vi "ScanningWaveformline_v1.vi"(0 "Vx-max":dbl, 1 "linepixels":dbl, 5 "Vx-min":dbl, 7 "AOrate":dbl, 9 "Vy-max":dbl, 11 "Vy-min":dbl, 12 "numlines":dbl) -> (3 "X-WaveArray":dbl[](array[numeric]), 6 "numPixels":dbl, 14 "Y-WaveArray":dbl[](array[numeric]), 15 "P":dbl)   [LabVIEW 2013]
panel:
  out "flyback time y (us)":dbl
  out "flyback time x (us)":dbl
  out "Waveform Graph 2":dbl[](graph)
  out "Waveform Graph":dbl[](graph)
  out "C":dbl
  out "S":dbl
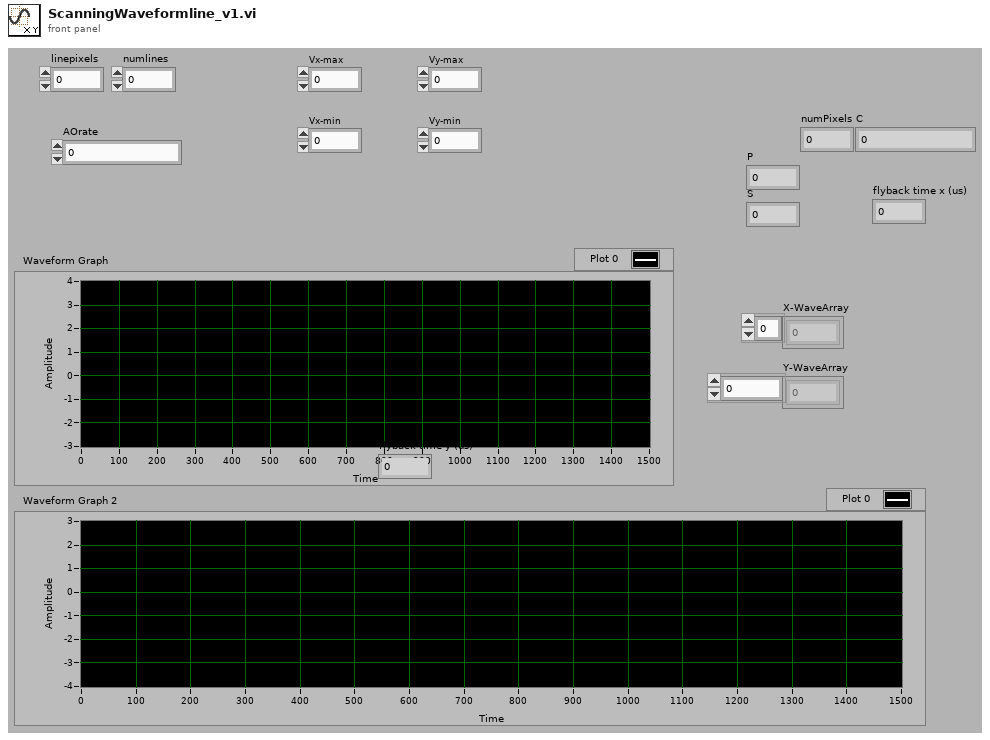
[diagram p1: front panel]
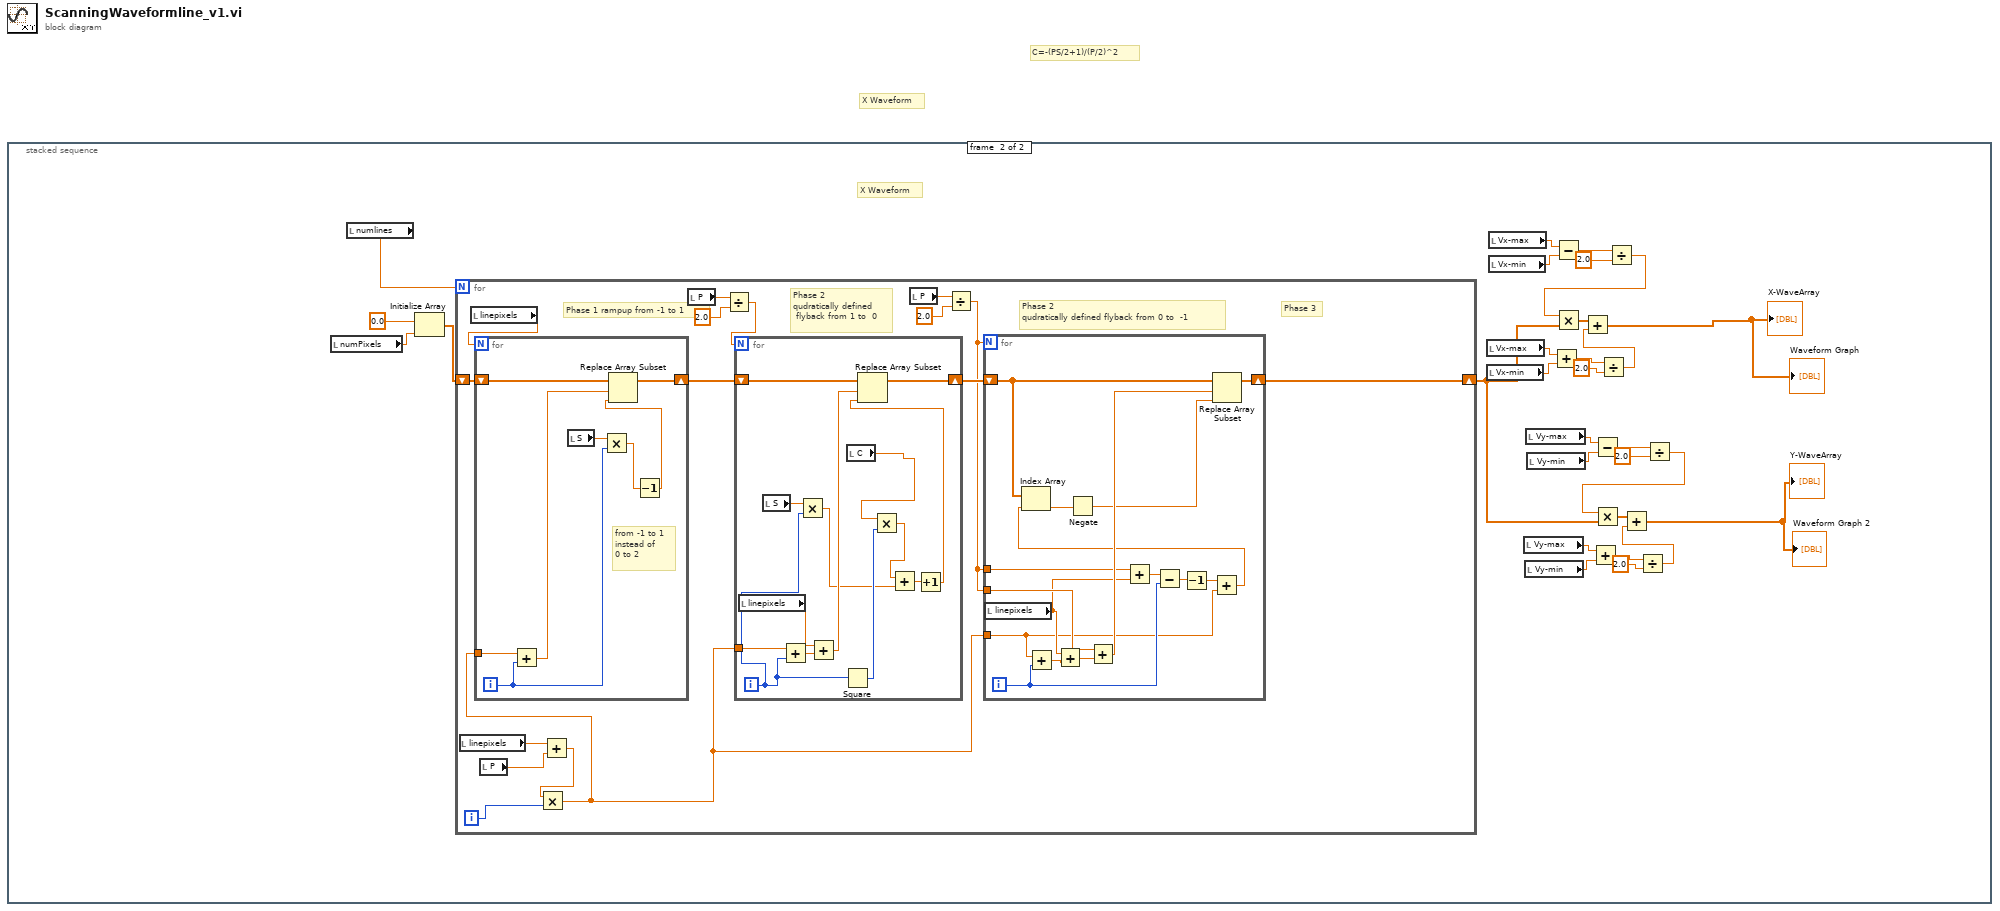
[diagram p0: block diagram]
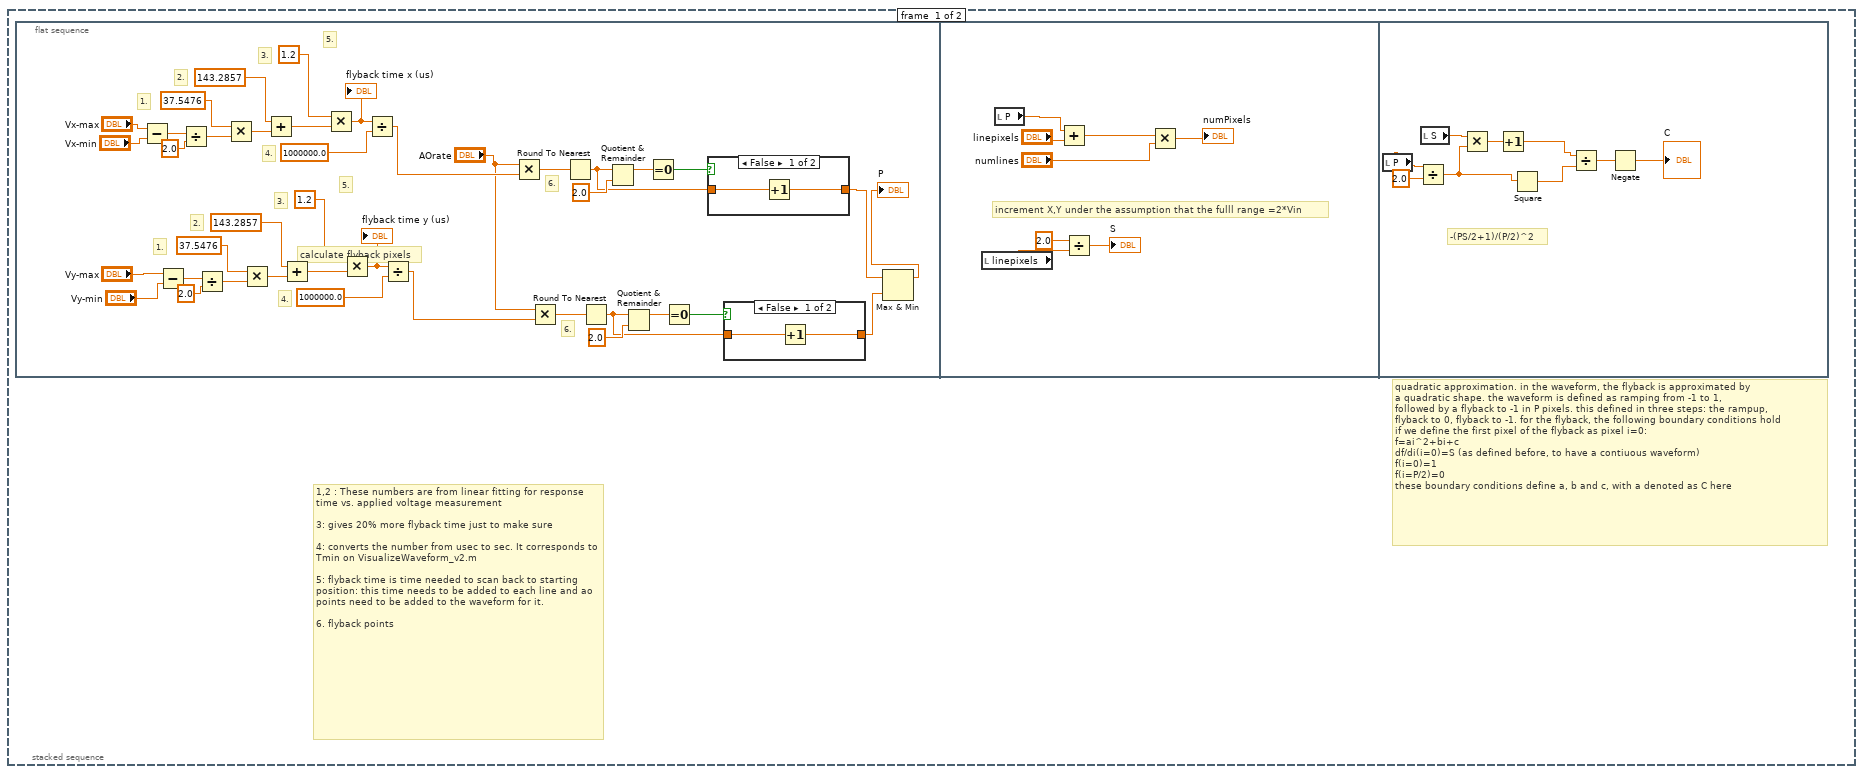
[diagram p2: hidden frame]
diagram:
  # "C=-(PS/2+1)/(P/2)^2"
  # "X Waveform"
  n1 = stacked-sequence {
    frame #0 {
      # "quadratic approximation. in the waveform, the flyback is approximated by\na quadratic shape. the waveform is defined as ramping from -1 to 1, \nfollowed by a flyback to -1 in P pixels. this defined in three steps: the rampup,\nflyback to 0, flyback to -1. for the flyback, the following boundary conditions hold\nif we define the first pixel of the flyback as pixel i=0:\nf=ai^2+bi+c\ndf/di(i=0)=S (as defined before, to have a contiuous waveform)\nf(i=0)=1\nf(i=P/2)=0\nthese boundary conditions define a, b and c, with a denoted as C here"
      # "1,2 : These numbers are from linear fitting for response time vs. applied voltage measurement\n\n3: gives 20% more flyback time just to make sure\n\n4: converts the number from usec to sec. It corresponds to Tmin on VisualizeWaveform_v2.m\n\n5: flyback time is time needed to scan back to starting position: this time needs to be added to each line and ao points need to be added to the waveform for it.\n\n6. flyback points"
      n2 = flat-sequence {
        frame #0 {
          # "6."
          # "5."
          # "4."
          # "3."
          # "2."
          # "1."
          # "calculate flyback pixels"
          # "6."
          # "5."
          # "4."
          # "3."
          # "2."
          # "1."
          n3 = Subtract(x="Vx-max", y="Vx-min") -> (x-y=w24:dbl)
          n4 = Subtract(x="Vy-max", y="Vy-min") -> (x-y=w8:dbl)
          n5 = Divide(x=w24, y=2.0 ("x-y")) -> (x/y=w23:dbl)
          n6 = Divide(x=w8, y=2.0 ("x-y")) -> (x/y=w7:dbl)
          n7 = Multiply(x=37.5476, y=w23) -> (x*y=w39:dbl)
          n8 = Multiply(x=37.5476, y=w7) -> (x*y=w21:dbl)
          n9 = Add(x=143.2857, y=w39) -> (x+y=w37:dbl)
          n10 = Add(x=143.2857, y=w21) -> (x+y=w19:dbl)
          n11 = Multiply(x=1.2, y=w37) -> (x*y=w35:dbl)
          "flyback time x (us)" <- w35
          n12 = Multiply(x=1.2, y=w19) -> (x*y=w17:dbl)
          "flyback time y (us)" <- w17
          n13 = Divide(x=w35, y=1000000.0 ("x")) -> (x/y=w33:dbl)
          n14 = Divide(x=w17, y=1000000.0 ("x")) -> (x/y=w15:dbl)
          n15 = Multiply(x="AOrate", y=w33) -> (x*y=w32:dbl)
          n16 = Multiply(x="AOrate", y=w15) -> (x*y=w14:dbl)
          n17 = Round To Nearest(number=w32) -> (nearest integer value=w28:dbl)
          n18 = Round To Nearest(number=w14) -> (nearest integer value=w10:dbl)
          n19 = Quotient & Remainder(x=w28, y=2.0) -> (x-y*floor(x/y)=w29:dbl)  [unwired: 1 out]
          n20 = Quotient & Remainder(x=w10, y=2.0) -> (x-y*floor(x/y)=w11:dbl)  [unwired: 1 out]
          n21 = Equal To 0?(x=w29) -> (x = 0?=w30:bool)
          n22 = Equal To 0?(x=w11) -> (x = 0?=w12:bool)
          n23 = case shown="False" w30 {
            tunnel: [w44 w46] -> w4
            tunnel: w28 -> [w45 w46]
            frame False {
              n24 = Increment(x=w45) -> (x+1=w44:dbl)
            }
            frame True {
            }
          }
          n25 = case shown="False" w12 {
            tunnel: [w41 w43] -> w5
            tunnel: w10 -> [w42 w43]
            frame False {
              n26 = Increment(x=w42) -> (x+1=w41:dbl)
            }
            frame True {
            }
          }
          n27 = Max & Min(x=w4, y=w5) -> (max(x,y)=→"P":dbl)  [unwired: 1 out]
        }
        frame #1 {
          # "increment X,Y under the assumption that the fulll range =2*Vin"
          n28 = local read "linepixels"() -> (w48:dbl)
          n29 = local read "P"() -> (w54:dbl)
          n30 = Add(x=w54, y="linepixels") -> (x+y=w50:dbl)
          n31 = Divide(x=2.0, y=w48) -> (x/y=→"S":dbl)
          n32 = Multiply(x=w50, y="numlines") -> (x*y=→"numPixels":dbl)
        }
        frame #2 {
          # "-(PS/2+1)/(P/2)^2"
          n33 = local read "P"() -> (w61:dbl)
          n34 = Divide(x=w61, y=2.0) -> (x/y=w63:dbl)
          n35 = local read "S"() -> (w62:dbl)
          n36 = Multiply(x=w62, y=w63) -> (x*y=w58:dbl)
          n37 = Increment(x=w58) -> (x+1=w55:dbl)
          n38 = Square(x=w63) -> (x^2=w59:dbl)
          n39 = Divide(x=w55, y=w59) -> (x/y=w60:dbl)
          n40 = Negate(x=w60) -> (-x=→"C":dbl)
        }
      }
    }
    frame #1 {
      # "X Waveform"
      n41 = local read "numPixels"() -> (w90:dbl)
      n42 = local read "numlines"() -> (w92:dbl)
      n43 = Initialize Array(0.0 ("element"), w90) -> (w89:dbl[])
      n44 = for {
        N: w92 -> [_]
        shift-right: [w94] -> w65
        shift-left: w89 -> [w103]
        i -> [w108]
        # "Phase 2\nqudratically defined flyback from 0 to  -1"
        # "Phase 3"
        # "Phase 2\nqudratically defined\n flyback from 1 to  0"
        # "Phase 1 rampup from -1 to 1"
        n45 = local read "linepixels"() -> (w107:dbl)
        n46 = local read "linepixels"() -> (w104:dbl)
        n47 = local read "P"() -> (w106:dbl)
        n48 = Add(x=w107, y=w106) -> (x+y=w105:dbl)
        n49 = Multiply(x=w105, y=w108) -> (x*y=w93:dbl)
        n50 = for {
          N: w104 -> [_]
          shift-right: [w140] -> w95
          shift-left: w103 -> [w146]
          tunnel: w93 -> [w139]
          i -> [w143]
          # "from -1 to 1\ninstead of\n0 to 2"
          n51 = Add(x=w139, y=w143) -> (x+y=w145:dbl)
          n52 = local read "S"() -> (w144:dbl)
          n53 = Multiply(x=w144, y=w143) -> (x*y=w142:dbl)
          n54 = Decrement(x=w142) -> (x-1=w141:dbl)
          n55 = Replace Array Subset(array=w146, new element=w141, index=w145) -> (w140:dbl[])
        }
        n56 = local read "P"() -> (w101:dbl)
        n57 = Divide(x=w101, y=2.0) -> (x/y=w102:dbl)
        n58 = for {
          N: w102 -> [_]
          shift-right: [w127] -> w97
          shift-left: w95 -> [w138]
          tunnel: w93 -> [w126]
          i -> [w131]
          n59 = local read "linepixels"() -> (w136:dbl)
          n60 = local read "S"() -> (w132:dbl)
          n61 = Add(x=w126, y=w131) -> (x+y=w137:dbl)
          n62 = Multiply(x=w132, y=w131) -> (x*y=w130:dbl)
          n63 = Add(x=w136, y=w137) -> (x+y=w135:dbl)
          n64 = Square(x=w131) -> (x^2=w134:i32)
          n65 = local read "C"() -> (w125:dbl)
          n66 = Multiply(x=w125, y=w134) -> (x*y=w133:dbl)
          n67 = Add(x=w133, y=w130) -> (x+y=w129:dbl)
          n68 = Increment(x=w129) -> (x+1=w128:dbl)
          n69 = Replace Array Subset(array=w138, new element=w128, index=w135) -> (w127:dbl[])
        }
        n70 = local read "P"() -> (w98:dbl)
        n71 = Divide(x=w98, y=2.0) -> (x/y=w96:dbl)
        n72 = for {
          N: w96 -> [_]
          tunnel: w96 -> [w122]
          tunnel: w96 -> [w119]
          shift-right: [w110] -> w94
          shift-left: w97 -> [w120]
          tunnel: w93 -> [w109]
          i -> [w116]
          n73 = local read "linepixels"() -> (w118:dbl)
          n74 = Add(x=w109, y=w116) -> (x+y=w124:dbl)
          n75 = Add(x=w118, y=w124) -> (x+y=w123:dbl)
          n76 = Add(x=w122, y=w123) -> (x+y=w121:dbl)
          n77 = Add(x=w119, y=w118) -> (x+y=w117:dbl)
          n78 = Subtract(x=w117, y=w116) -> (x-y=w115:dbl)
          n79 = Decrement(x=w115) -> (x-1=w114:dbl)
          n80 = Add(x=w114, y=w109) -> (x+y=w113:dbl)
          n81 = Index Array(array=w120, index=w113) -> (element=w112:dbl)
          n82 = Negate(x=w112) -> (-x=w111:dbl)
          n83 = Replace Array Subset(array=w120, new element=w111, index=w121) -> (w110:dbl[])
        }
      }
      n84 = local read "Vx-max"() -> (w81:dbl)
      n85 = local read "Vx-min"() -> (w80:dbl)
      n86 = local read "Vx-max"() -> (w84:dbl)
      n87 = local read "Vx-min"() -> (w85:dbl)
      n88 = local read "Vy-max"() -> (w72:dbl)
      n89 = local read "Vy-min"() -> (w73:dbl)
      n90 = local read "Vy-max"() -> (w70:dbl)
      n91 = local read "Vy-min"() -> (w69:dbl)
      n92 = Add(x=w81, y=w80) -> (x+y=w79:dbl)
      n93 = Subtract(x=w84, y=w85) -> (x-y=w86:dbl)
      n94 = Add(x=w72, y=w73) -> (x+y=w74:dbl)
      n95 = Subtract(x=w70, y=w69) -> (x-y=w68:dbl)
      n96 = Divide(x=w79, y=2.0) -> (x/y=w77:dbl)
      n97 = Divide(x=w86, y=2.0) -> (x/y=w83:dbl)
      n98 = Multiply(x=w83, y=w65) -> (x*y=w88:dbl[])
      n99 = Add(x=w88, y=w77) -> (x+y=→"X-WaveArray" →"Waveform Graph":dbl[])
      n100 = Divide(x=w74, y=2.0) -> (x/y=w76:dbl)
      n101 = Divide(x=w68, y=2.0) -> (x/y=w71:dbl)
      n102 = Multiply(x=w71, y=w65) -> (x*y=w66:dbl[])
      n103 = Add(x=w66, y=w76) -> (x+y=→"Y-WaveArray" →"Waveform Graph 2":dbl[])
    }
  }
